vi "Init.vi"(8 "error in (no error)":errorcluster, 10 "Instrument Interface":refnum<class "Instrument.lvclass">, 11 "Low Level PSU In":refnum<class "Low Level PSU.lvclass">) -> (0 "error out":errorcluster, 3 "Low Level PSU Out":refnum<class "Low Level PSU.lvclass">)   [LabVIEW 2020, in "Low Level PSU With Tests.lvlib" / "Low Level PSU.lvclass"]
uses:
  Low Level PSU.lvclass
  Instrument Interface/Instrument.lvclass
  Low Level PSU.lvclass/Low Level PSU.ctl
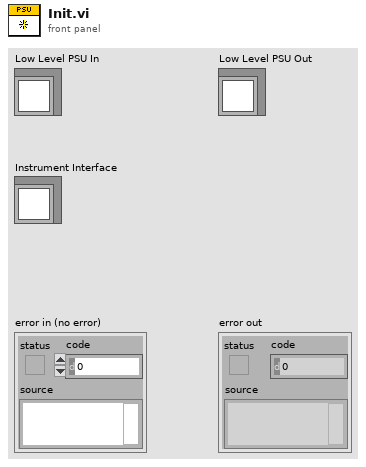
[diagram p1: front panel]
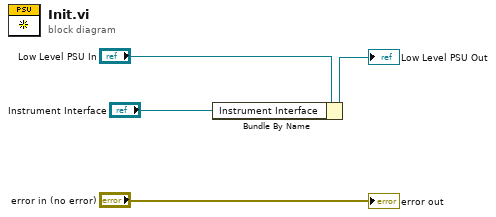
[diagram p0: block diagram]
diagram:
  n1 = Bundle By Name(cluster="Low Level PSU In", "Instrument Interface"="Instrument Interface") -> (→"Low Level PSU Out":refnum<class "Low Level PSU.lvclass">)
  "error out" <- "error in (no error)"
